vi "ADC debug (RT).vi"() -> ()   [LabVIEW 2019]
uses:
  <vilib>/rvi/interface/nirviOpenFPGA/nirviOpenFPGA.xnode
  FPGA Bitfiles/tisbrio_FPGATarget(9626)_ADCdebug_yznjIum4Ycg.lvbitx
  <vilib>/rvi/interface/nirviReadWriteControl/nirviReadWriteControl.xnode
  <vilib>/rvi/interface/nirviCloseFPGA/nirviCloseFPGA.xnode
  <vilib>/FPGAPlugInAG/sbRIO-9626/niLvFpga_Close_sbRIO-9626.vi
  <vilib>/rvi/errors/niLvFpgaAdjustHostInterfaceError.vi
  <vilib>/FPGAPlugInAG/sbRIO-9626/niLvFpga_Open_sbRIO-9626.vi
  <vilib>/rvi/errors/niLvFpgaMergeErrorWithErrorCode.vi
  NiFpgaLv.dll
  <vilib>/Utility/error.llb/Error Cluster From Error Code.vi
panel:
  out "Waveform Chart":dbl(graph)
  out "AI16-47":fxp<+/-,28,17>[](array[numeric])
  in  "stop":bool
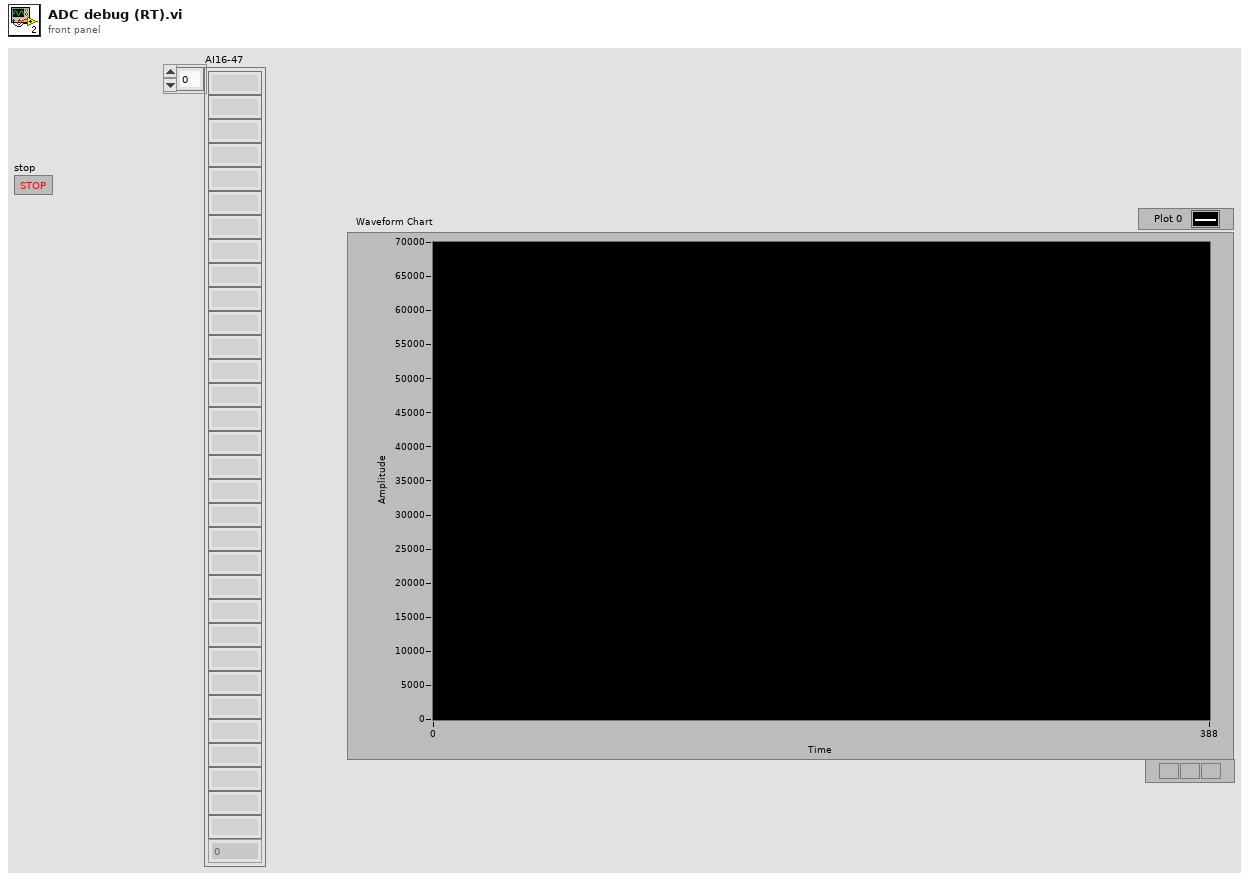
[diagram p1: front panel]
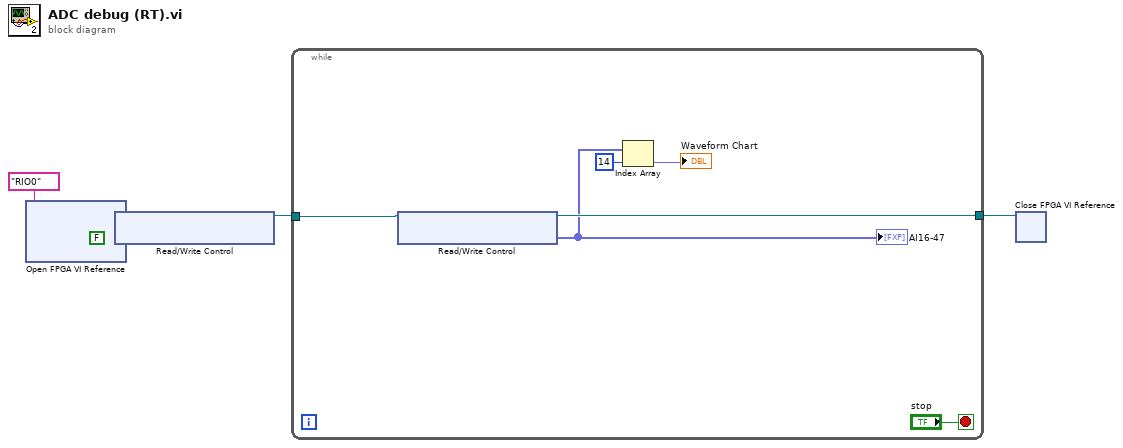
[diagram p0: block diagram]
diagram:
  n1 = xnode "Open FPGA VI Reference"("resource name"=tag "RIO0") -> ("FPGA VI Reference Out"=w3:refnum<k20>)  [unwired: 1 in, 1 out]
  n2 = xnode "Read/Write Control"("FPGA VI Reference In"=w3, "Auto Reset"=FALSE) -> ("FPGA VI Reference Out"=w2:refnum<k20>)  [unwired: 1 in, 1 out]
  n3 = while {
    tunnel: w2 -> [w9]
    tunnel: [w10] -> w4
    stop <- "stop" stop-if-true
    n4 = xnode "Read/Write Control"("FPGA VI Reference In"=w9) -> ("FPGA VI Reference Out"=w10:refnum<k20>, "AI16-47"=w8:fxp<+/-,28,17>[])  [unwired: 1 in, 1 out]
    "AI16-47" <- w8
    n5 = Index Array(array=w8, index=14) -> (element=→"Waveform Chart":fxp<+/-,28,17>)
  }
  n6 = xnode "Close FPGA VI Reference"("FPGA VI Reference In"=w4) -> ()  [unwired: 1 in, 1 out]
